vi "Tosca-DI Write Thread.vi"(0 "Write Data":refnum<queue>, 5 "IPC":T1, 9 "Digital Inputs":T6[](array[typedef]), 11 "Input Events":T2[](array[typedef])) -> (4 "Write Data thru":refnum<queue>, 15 "error out":errorcluster)   [LabVIEW 2020]
uses:
  Tosca-Digital Input.ctl
  Tosca-Input Event.ctl
  Tosca-Input Criterion.ctl
  epl-vi-lib/Utility VIs/Type Defs/Logic State.ctl
  Typedefs/Tosca-Accumulator.ctl
  Tosca-DI Write Data.ctl
  IPC VIs/Tosca-IPC.ctl
  Classes/Parameters/Parameters.lvclass
  Tosca-DI Queue Data.ctl
  Typedefs/Tosca-State AODO.ctl
  Typedefs/Tosca-AO Runtime.ctl
  Typedefs/Tosca-DO Runtime.ctl
  epl-vi-lib/Signal Synthesis VIs/4th Generation/Classes/SignalManager/SignalManager.lvclass
  Typedefs/Tosca-Synapse Start Data.ctl
  IPC VIs/Tosca-Message.ctl
  IPC VIs/Tosca-Message Action.ctl
  Typedefs/Tosca-Thread Type.ctl
  Imaging VIs/Tosca-2P-Notifier Data.ctl
  Typedefs/Tosca-MATLAB Queue Data.ctl
  Visual Stim VIs/Tosca-Grating.ctl
  Visual Stim VIs/Tosca-Grating Type.ctl
  Typedefs/Tosca-File IO Notification.ctl
  epl-vi-lib/Utility VIs/Controls/Utilities-Wait.vi/89bc9713-8f2c-40bd-a11f-1c800a437687.vi
  <vilib>/Utility/error.llb/Error Cluster From Error Code.vi
  <vilib>/Utility/High Resolution Polling Wait.vi
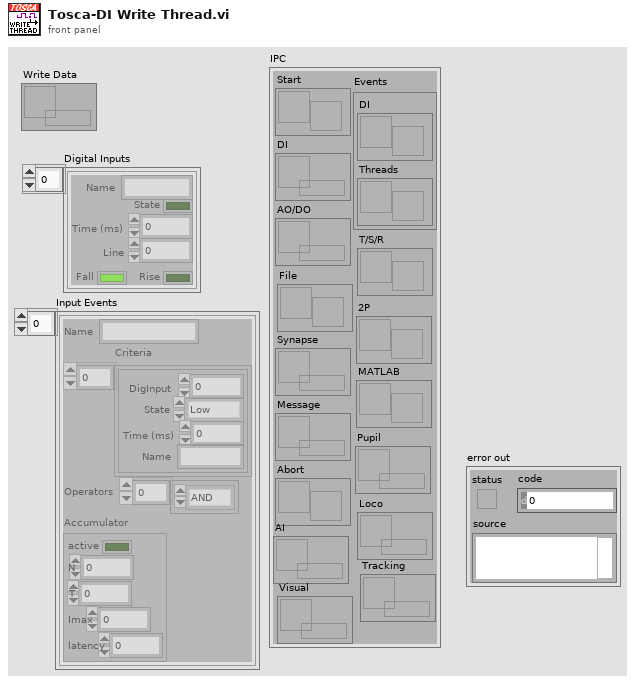
[diagram p1: front panel]
types:
  T1 = typedef "Tosca-IPC.ctl" = cluster{"Start":refnum<notifier>, "DI":refnum<queue>, "AO/DO":refnum<queue>, "Synapse":refnum<queue>, "Message":refnum<queue>, "Abort":refnum<notifier>, "Events":cluster{"DI":refnum<user-event>, "Threads ":refnum<user-event>}, "T/S/R":refnum<notifier>, "2P":refnum<notifier>, "MATLAB":refnum<notifier>, "Pupil":refnum<queue>, "Loco":refnum<queue>, "AI":refnum<queue>, "Tracking":refnum<queue>, "Visual":refnum<queue>, "File":refnum<notifier>}
  T2 = typedef "Tosca-Input Event.ctl" = cluster{"Name":string, "Criteria":T3[], "Operators":enum16{"AND", "OR"}[], "Accumulator":T5}
  T3 = typedef "Tosca-Input Criterion.ctl" = cluster{"DigInput":i32, "State":T4, "Time (ms)":i32, "Name":string}
  T4 = typedef "Logic State.ctl" = enum16{"Low", "High", "Rising", "Falling"}
  T5 = typedef "Tosca-Accumulator.ctl" = cluster{"active":bool, "N":i32, "T":dbl, "Imax":dbl, "latency":dbl}
  T6 = typedef "Tosca-Digital Input.ctl" = cluster{"Name":string, "State":bool, "Time (ms)":dbl, "Line":i32, "Rise":bool, "Fall":bool}
  T7 = typedef "Tosca-DI Write Data.ctl" = cluster{"loop time":dbl, "digital":bool[], "events":bool[], "last":bool, "time":dbl}
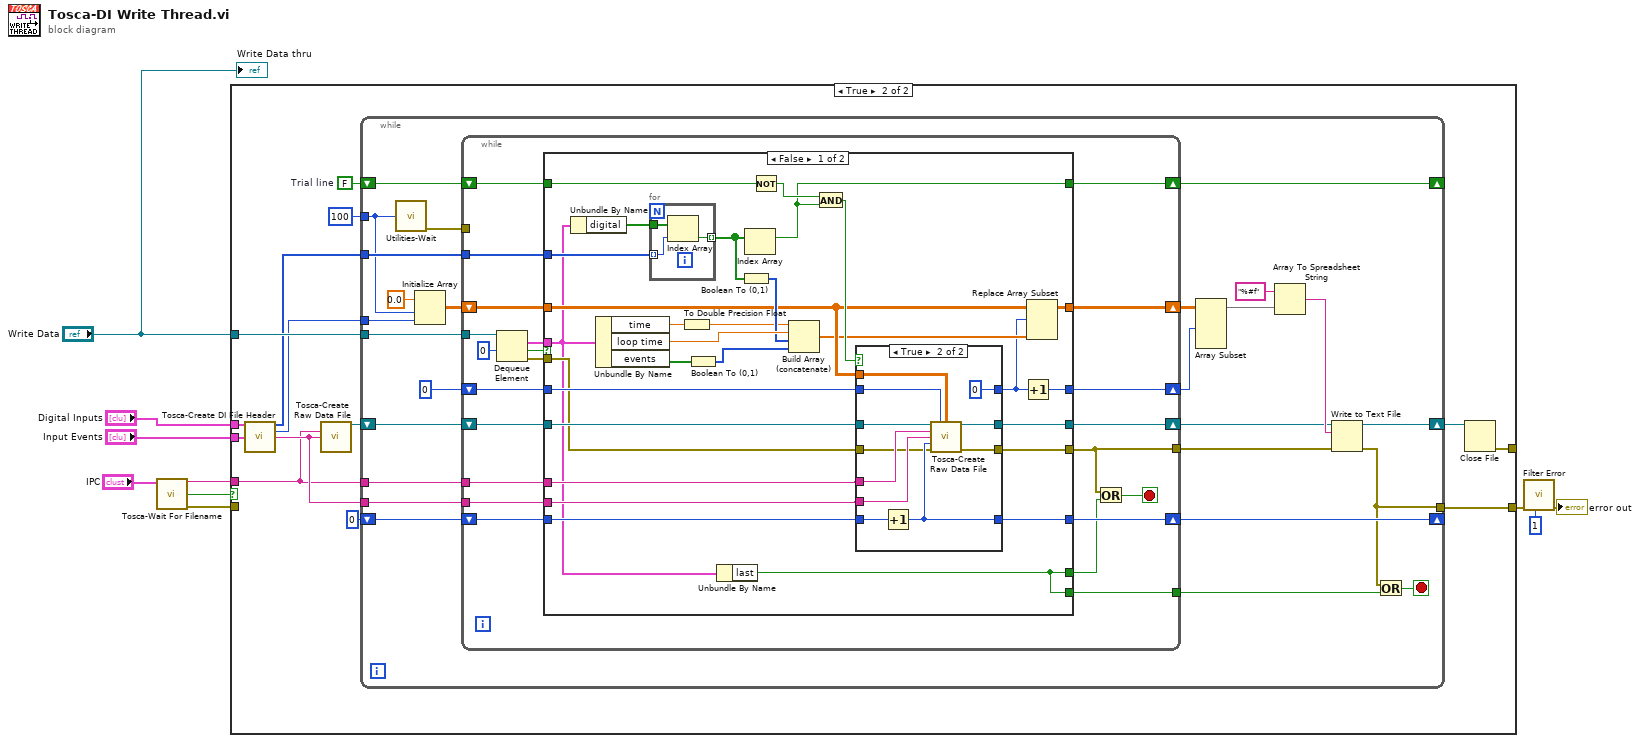
[diagram p0: block diagram]
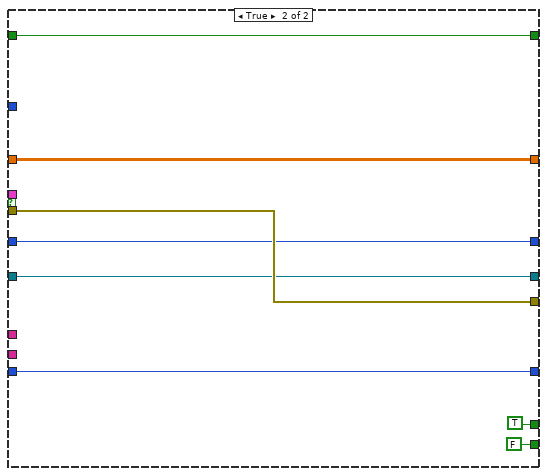
[diagram p4: hidden frame]
diagram:
  n1 = call "Tosca-Wait For Filename.vi"("IPC"="IPC") -> ("Filestem"=w4:string, "Received"=w3:bool, "error out"=w2:errorcluster)  [unwired: 12 in]
  n2 = case shown="True" w3 {
    tunnel: [w11 w23] -> w10
    tunnel: "Write Data" -> [_ w20]
    tunnel: "Digital Inputs" -> [_ w18]
    tunnel: "Input Events" -> [_ w17]
    tunnel: w4 -> [_ w13]
    tunnel: w2 -> [w11 _]
    tunnel: [_ w12] -> _
    frame False {
    }
    frame True {
      w22 = FALSE  # Trial line
      n3 = call "Tosca-Create DI File Header.vi"("Digital Inputs"=w18, "Input Events"=w17) -> ("DI Write Order"=w16:i32[], "Num Columns"=w15:i32, "header"=w19:string)  [unwired: 11 in]
      n4 = call "Tosca-Create Raw Data File.vi"("Filestem"=w13, "Header"=w19) -> ("refnum out"=w21:refnum<file>)  [unwired: 12 in, 1 out]
      n5 = while {
        tunnel: u32 100 -> [w30]
        shift-right: [w50] -> _
        shift-left: 0 -> [w51]
        tunnel: w20 -> [w48]
        tunnel: [w38] -> w23
        shift-right: [w46] -> _
        shift-left: w22 -> [w47]
        shift-right: [w31] -> w14
        shift-left: w21 -> [w40]
        tunnel: w16 -> [w45]
        tunnel: w13 -> [w37]
        tunnel: w19 -> [w36]
        tunnel: w15 -> [w29]
        stop <- w49 stop-if-true
        n6 = call "Utilities-Wait.vi"("milliseconds to wait"=w30) -> ("error out"=w33:errorcluster)  [unwired: 14 in]
        n7 = Initialize Array(0.0 ("element"), w30, w29) -> (w42:dbl[][])
        n8 = while {
          shift-right: [w57] -> w50
          shift-left: w51 -> [w58]
          tunnel: w48 -> [w73]
          shift-right: [w68] -> w46
          shift-left: w47 -> [w69]
          tunnel: w45 -> [w66]
          shift-right: [w61] -> w27
          shift-left: 0 -> [w65]
          shift-right: [w56] -> w41
          shift-left: w42 -> [w64]
          shift-right: [w62] -> w32
          shift-left: w40 -> [w63]
          tunnel: w37 -> [w60]
          tunnel: w36 -> [w59]
          tunnel: [w55] -> w35
          tunnel: [w52] -> w34
          tunnel: w33 -> [_]
          stop <- w53 stop-if-true
          n9 = Dequeue Element(queue=w73, timeout in ms (-1)=0) -> (element=w71:T7, timed out?=w67:bool, error out=w72:errorcluster)  [unwired: 1 in, 1 out]
          n10 = case shown="False" w67 {
            tunnel: w72 -> [w81 w126]
            tunnel: w71 -> [w79 _]
            tunnel: w69 -> [w101 w128]
            tunnel: [w98 w128] -> w68
            tunnel: w66 -> [w99 _]
            tunnel: w64 -> [w84 w127]
            tunnel: w65 -> [w95 w125]
            tunnel: w63 -> [w90 w124]
            tunnel: [w89 w124] -> w62
            tunnel: [w77 w125] -> w61
            tunnel: w60 -> [w88 _]
            tunnel: w59 -> [w87 _]
            tunnel: w58 -> [w86 w123]
            tunnel: [w85 w123] -> w57
            tunnel: [w82 w127] -> w56
            tunnel: [w80 w126] -> w55
            tunnel: [w76 TRUE ("last")] -> w54
            tunnel: [w76 FALSE ("last")] -> w52
            frame False {
              n11 = Unbundle By Name(w79) -> ("digital"=w102:bool[])
              n12 = Unbundle By Name(w79) -> ("time"=w75:dbl, "loop time"=w94:dbl, "events"=w97:bool[])
              n13 = for {
                tunnel: w102 -> [w120]
                tunnel: [w119] -> w96 mode=indexing
                tunnel: w99 -> [w118] mode=indexing
                n14 = Index Array(array=w120, index=w118) -> (element=w119:bool)
              }
              n15 = To Double Precision Float(number=w75) -> (double precision float=w74:dbl)
              n16 = Boolean To (0,1)(Boolean=w97) -> (0, 1=w92:i16[])
              n17 = Unbundle By Name(w79) -> ("last"=w76:bool)
              n18 = Boolean To (0,1)(Boolean=w96) -> (0, 1=w93:i16[])
              n19 = Index Array(array=w96) -> (element=w98:bool)  [unwired: 1 in]
              n20 = Not(x=w101) -> (.not. x?=w100:bool)
              n21 = Build Array (concatenate)(w74, w94, w93, w92) -> (w83:dbl[])
              n22 = And(x=w100, y=w98) -> (x .and. y?=w91:bool)
              n23 = case shown="True" w91 {
                tunnel: w95 -> [w104 w107]
                tunnel: w90 -> [w106 w117]
                tunnel: [w106 w116] -> w89
                tunnel: [w104 0] -> w78
                tunnel: w88 -> [_ w115]
                tunnel: w87 -> [_ w114]
                tunnel: w86 -> [w105 w113]
                tunnel: [w105 w112] -> w85
                tunnel: w84 -> [_ w108]
                tunnel: w81 -> [w103 w110]
                tunnel: [w103 w109] -> w80
                frame False {
                }
                frame True {
                  n24 = Increment(x=w113) -> (x+1=w112:i32)
                  n25 = call "Tosca-Create Raw Data File.vi"("refnum in"=w117, "Length"=w107, "Remainder"=w108, "Filestem"=w115, "Header"=w114, "Trial Number"=w112, "error in"=w110) -> ("refnum out"=w116:refnum<file>, "error out"=w109:errorcluster)  [unwired: 7 in]
                }
              }
              n26 = Increment(x=w78) -> (x+1=w77:i32)
              n27 = Replace Array Subset(array=w84, new element=w83, index (row)=w78) -> (w82:dbl[][])  [unwired: 1 in]
            }
            frame True {
            }
          }
          n28 = Or(x=w55, y=w54) -> (x .or. y?=w53:bool)
        }
        n29 = Array Subset(array=w41, length (row)=w27) -> (w28:dbl[][])  [unwired: 3 in]
        n30 = Array To Spreadsheet String(array=w28, 3:"%#f" ("format string")) -> (spreadsheet string=w39:string)  [unwired: 1 in]
        n31 = Write to Text File(file (use dialog)=w32, text=w39, error in=w35) -> (refnum out=w31:refnum<file>, error out=w38:errorcluster)  [unwired: 1 in, 1 out]
        n32 = Or(x=w38, y=w34) -> (x .or. y?=w49:bool)
      }
      n33 = Close File(refnum=w14) -> (error out=w12:errorcluster)  [unwired: 1 in, 1 out]
    }
  }
  n34 = call "Filter Error.vi"("error in (no error)"=w10, "code to ignore"=1) -> ("error out"=→"error out":errorcluster)  [unwired: 9 in]
  "Write Data thru" <- "Write Data"
